vi "UpgradeFirmware_Main.vi"(8 "error in (no error)":errorcluster, 11 "DevInfo":T1={"Hostname"="", "IPAddress"="", "MAC"="", "SerialNum"="", "Model"="", "Status"="", "FW"="", "OSDesc"="", "ImgTitle"="", "ImgDesc"="", "ImgVer"="", "ImgID"="", "IP Address Request Mode"=1, "SubnetMask"="", "Gateway"="", "DNSServer"=""} {"IP Address Request Mode" items=["Static"=1, "DHCP/Link-Local"=2, "Link-Local Only"=4, "DHCP Only"=8]}) -> (0 "error out":errorcluster)   [LabVIEW 2021]
uses:
  TypeDefs/DevInfo.ctl
  TypeDefs/DeployImageStates.ctl
  TypeDefs/AppImageProperties.ctl
  TypeDefs/FPGA_Properties_Element.ctl
  <vilib>/Utility/config.llb/Read Key (String).vi
  <vilib>/Utility/config.llb/NI_LVConfig.lvlib
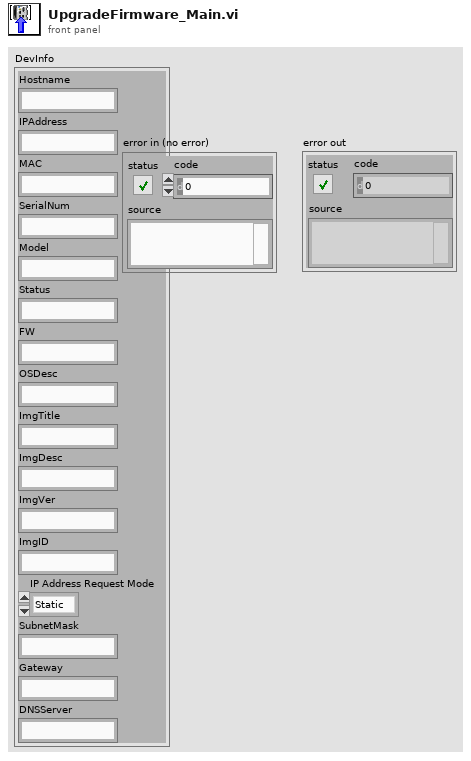
[diagram p1: front panel]
types:
  T1 = typedef "DevInfo.ctl" = cluster{"Hostname":string, "IPAddress":string, "MAC":string, "SerialNum":string, "Model":string, "Status":string, "FW":string, "OSDesc":string, "ImgTitle":string, "ImgDesc":string, "ImgVer":string, "ImgID":string, "IP Address Request Mode":i32, "SubnetMask":string, "Gateway":string, "DNSServer":string}
  T2 = typedef "AppImageProperties.ctl" = cluster{"Name":string, "Version":string, "Time":timestamp, "Description":string, "Key":string, "Chassis":string, "FPGA Properties":T3[], "Model":string, "Retrieve":string[], "Deploy":string[], "Installed Software":string[]}
  T3 = typedef "FPGA_Properties_Element.ctl" = cluster{"Resource Name":string, "Path":path}
  T4 = typedef "DeployImageStates.ctl" = enum16{"Select Image File", "Extract Image", "Display Image Info", "Deploy Image", "Clean Up", "Exit"}
  T5 = cluster{"Selected Image File":path, "AppImage Properties":T2}
  T6 = typedef "NI_LVConfig.lvlib/Config Data RefNum.ctl" = refnum<k1>
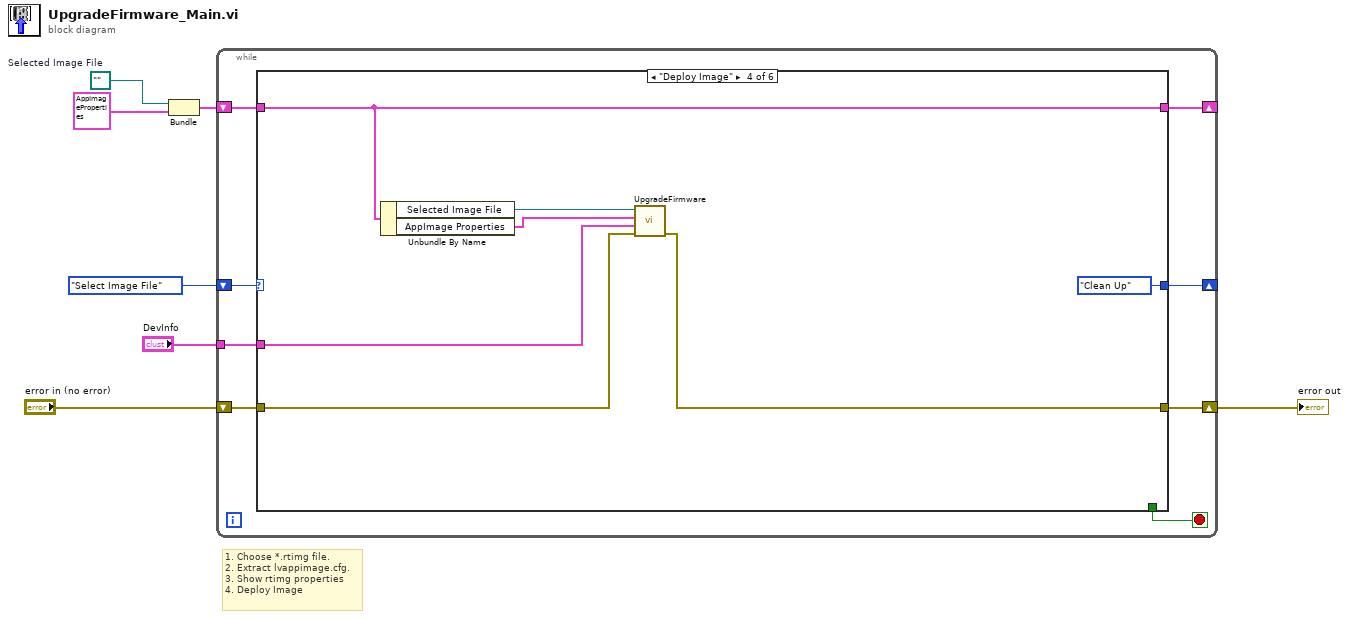
[diagram p0: block diagram]
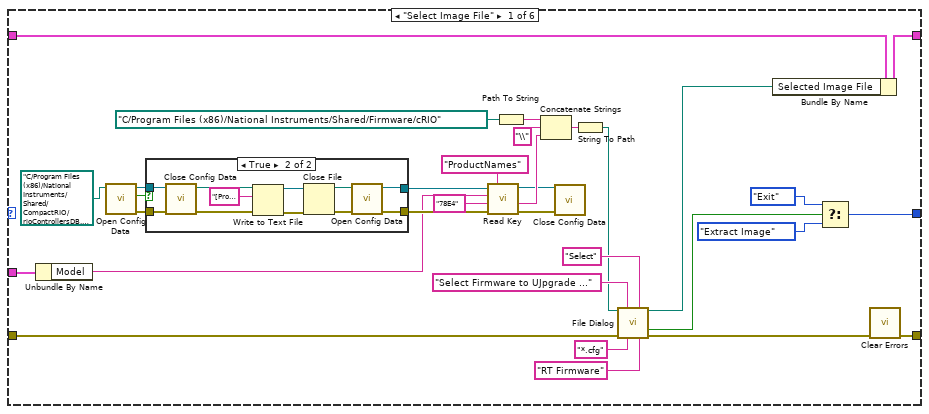
[diagram p2: hidden frame]
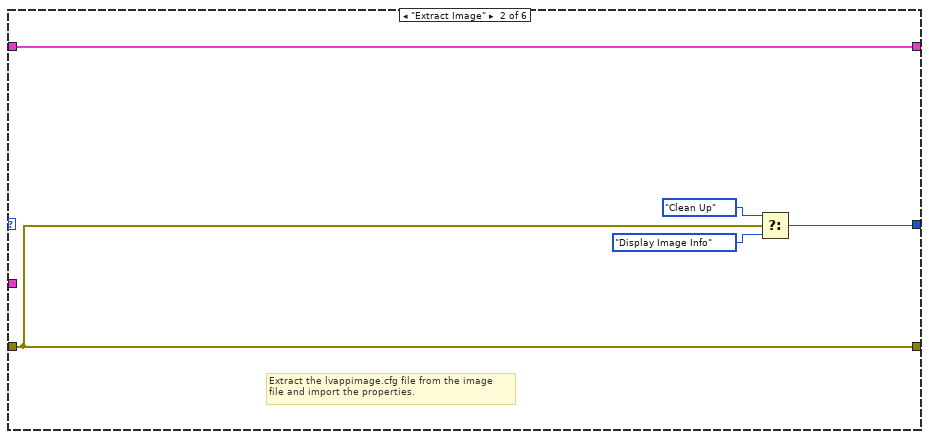
[diagram p4: hidden frame]
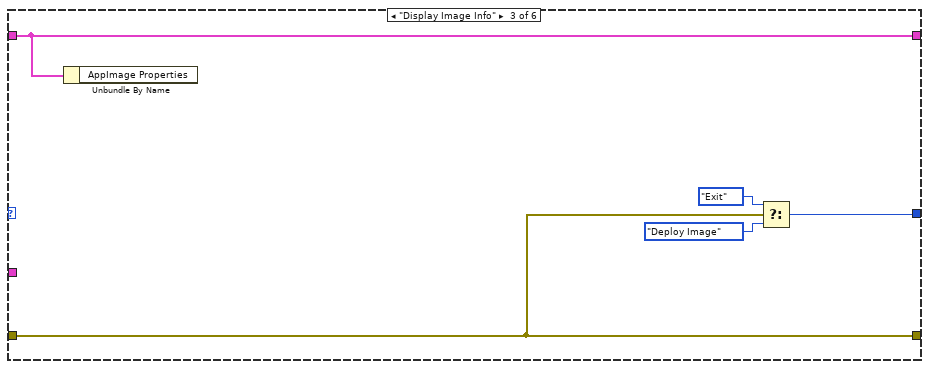
[diagram p5: hidden frame]
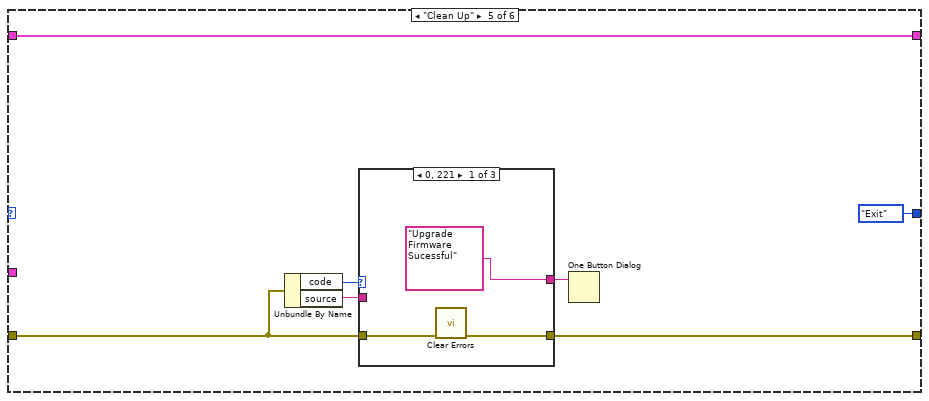
[diagram p6: hidden frame]
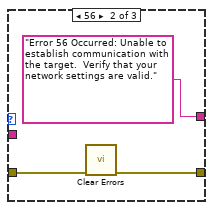
[diagram p7: hidden frame]
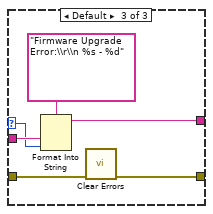
[diagram p8: hidden frame]
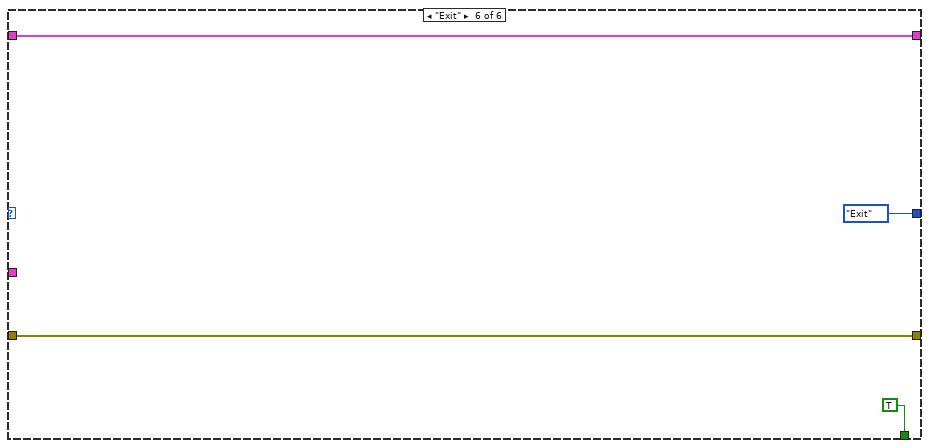
[diagram p9: hidden frame]
diagram:
  w4 = path ""  # Selected Image File
  # "1. Choose *.rtimg file.\n2. Extract lvappimage.cfg.\n3. Show rtimg properties\n4. Deploy Image"
  n1 = Bundle("Selected Image File"=w4, "AppImage Properties"=T2 {"Name"="", "Version"="", "Time"=timestamp(0 s since 1904-01-01), "Description"="", "Key"="", "Chassis"="", "FPGA Properties"=[], "Model"="", "Retrieve"=[], "Deploy"=[], "Installed Software"=[]}) -> (w3:T5)  [unwired: 1 in]
  n2 = while {
    shift-right: [w12] -> _
    shift-left: DeployImageStates."Select Image File" -> [w15]
    shift-right: [w13] -> w5
    shift-left: "error in (no error)" -> [w14]
    shift-right: [w10] -> _
    shift-left: w3 -> [w11]
    tunnel: "DevInfo" -> [w8]
    stop <- w9 stop-if-true
    n3 = case shown="\"Deploy Image\"" w15 {
      tunnel: w14 -> [w44 w65 w66 w72 w81 w98]
      tunnel: [w38 w65 w66 w71 w80 w98] -> w13
      tunnel: [w40 w61 w68 DeployImageStates."Clean Up" DeployImageStates."Exit" DeployImageStates."Exit"] -> w12
      tunnel: w11 -> [w34 w64 w67 w76 w79 w99]
      tunnel: [w37 w64 w67 w76 w79 w99] -> w10
      tunnel: [_ _ _ _ _ TRUE] -> w9
      tunnel: w8 -> [w17 _ _ w73 _ _]
      frame "Select Image File" {
        n4 = Unbundle By Name(w17) -> ("Model"=w16:string)
        n5 = call <vilib>:"Open Config Data.vi"("configuration file path"=path "C:/Program Files (x86)/National Instruments/Shared/CompactRIO/rioControllersDB.ini" ("start path")) -> ("error out"=w27:errorcluster, "file created?"=w25:bool, "refnum"=w26:T6)  [unwired: 8 in]
        n6 = case shown="True" w25 {
          tunnel: w26 -> [w49 w60]
          tunnel: w27 -> [w48 w59]
          tunnel: [w49 w54] -> w28
          tunnel: [w48 w50] -> w29
          frame False {
          }
          frame True {
            n7 = call <vilib>:"Close Config Data.vi"("error in (no error)"=w59, "refnum"=w60) -> ("error out"=w52:errorcluster, "file path"=w58:path)  [unwired: 8 in]
            n8 = Write to Text File(file (use dialog)=w58, text="[ProductNames]\nsbRIO-9601=7373\nsbRIO-9602=7373\nsbRIO-9611=7373\nsbRIO-9612=7373\nsbRIO-9631=7373\nsbRIO-9632=7373\nsbRIO-9641=7373\nsbRIO-9642=7373\nsbRIO-9605=758B\nsbRIO-9606=758B\nsbRIO-9623=758B\nsbRIO-9626=758B\nsbRIO-9633=758B\nsbRIO-9636=758B\nsbRIO-9651=775E\nsbRIO-9607=77D6\nsbRIO-9627=77D5\nsbRIO-9637=77D4\nsbRIO-9603=7A38\nsbRIO-9608=7A39\nsbRIO-9609=7A41\nsbRIO-9628=7A3A\nsbRIO-9629=7A43\nsbRIO-9638=7A3B\n\ncRIO-9002=705F\ncRIO-9004=705F\ncRIO-9012=718F\ncRIO-9014=7319\ncRIO-9022=73D2\ncRIO-9023=73D2\ncRIO-9024=7459\ncRIO-9025=7459\ncRIO-9030=7755\ncRIO-9031=774B\ncRIO-9032=7841\ncRIO-9033=7735\ncRIO-9034=774D\ncRIO-9035=77DB\ncRIO-9035 (Sync)=7875\ncRIO-9036=77DC\ncRIO-9037=7840\ncRIO-9038=77B9\ncRIO-9039=77DD\ncRIO-9039 (Sync)=7878\ncRIO-9040=78E3\ncRIO-9041=79D0\ncRIO-9042=78E8\ncRIO-9043=78E5\ncRIO-9045=78E4\ncRIO-9046=79CE\ncRIO-9047=78E9\ncRIO-9048=78B7\ncRIO-9048 (TPM)=78E7\ncRIO-9049=78EA\ncRIO-9053=79DD\ncRIO-9054=79DE\ncRIO-9055=7A2B\ncRIO-9056=79DF\ncRIO-9057=79E0\ncRIO-9058=7A2A\ncRIO-9072=71C7\ncRIO-9073=71C7\ncRIO-9074=729D\ncRIO-9075=7527\ncRIO-9076=7527\ncRIO-9081=753D\ncRIO-9082=753D\ncRIO-9081_$$=751A\ncRIO-9082_$$=751A\ncRIO-9063=7740\ncRIO-9064=7741\ncRIO-9065=7742\ncRIO-9066=7743\ncRIO-9067=7744\ncRIO-9068=76D6\n\nNI 9146=75C8\nNI 9147=774C\nNI 9148=74E8\nNI 9149=774E\n\nmyRIO-1900=762F\nmyRIO-1950=76D3\nroboRIO=76F2\nroboRIO 2.0=7AAE\nELVIS RIO CM=7885\nELVIS III=793C\n\ncRIO-9081_$$_$$=753D_2\ncRIO-9082_$$_$$=753D_2\n\n; lvRioProviderVersion is Major*1000000 + Minor*1000 + Update\n[LabVIEWSupportRemoved_lvRioProviderVersion]\ncRIO-9002=17000000\ncRIO-9004=17000000\ncRIO-9072=17000000\ncRIO-9012=19000000\ncRIO-9014=19000000\ncRIO-9022=20000000\ncRIO-9023=20000000\ncRIO-9024=20000000\ncRIO-9025=20000000\ncRIO-9072=20000000\ncRIO-9073=20000000\ncRIO-9074=20000000\ncRIO-9075=20000000\ncRIO-9076=20000000\ncRIO-9081=20000000\ncRIO-9082=20000000\ncRIO-9081_$$=20000000\ncRIO-9082_$$=20000000\ncRIO-9081_$$_$$=20000000\ncRIO-9082_$$_$$=20000000\nsbRIO-9601=20000000\nsbRIO-9602=20000000\nsbRIO-9611=20000000\nsbRIO-9612=20000000\nsbRIO-9631=20000000\nsbRIO-9632=20000000\nsbRIO-9641=20000000\nsbRIO-9642=20000000\nsbRIO-9605=20000000\nsbRIO-9606=20000000\nsbRIO-9623=20000000\nsbRIO-9626=20000000\nsbRIO-9633=20000000\nsbRIO-9636=20000000\nNI 9146=20000000\nNI 9148=20000000\n\n[7373]\nsupportChassisAddition_lvRioProviderVersion=14000000\nsupportedInLabVIEW_lvRioProviderVersion=13000000\nproductLine=sbRIO\npngIcon16=SingleBoardRIOController.png\npngWarningIcon16=SingleBoardRIOControllerWarning.png\noperatingSystem=vxworks\ncpuArchitecture=ppc\nmonolithic=true\nsupportsRsi_lvRioProviderVersion=13000000\n\n[758B]\nsupportChassisAddition_lvRioProviderVersion=14000000\nsupportedInLabVIEW_lvRioProviderVersion=13000000\nproductLine=sbRIO\npngIcon16=SingleBoardRIOController.png\npngWarningIcon16=SingleBoardRIOControllerWarning.png\noperatingSystem=vxworks\ncpuArchitecture=ppc\nmonolithic=true\nneedsDDPSwitches=true\nsupportsRsi_lvRioProviderVersion=13000000\n\n[705F]\nsupportChassisAddition_lvRioProviderVersion=14000000\nsupportedInLabVIEW_lvRioProviderVersion=13000000\nproductLine=cRIO\npngIcon16=CompactRIOController.png\npngWarningIcon16=CompactRIOControllerWarning.png\noperatingSystem=pharlap\ncpuArchitecture=x86\n\n[718F]\nsupportChassisAddition_lvRioProviderVersion=14000000\nsupportedInLabVIEW_lvRioProviderVersion=13000000\nproductLine=cRIO\npngIcon16=CompactRIOController.png\npngWarningIcon16=CompactRIOControllerWarning.png\noperatingSystem=vxworks\ncpuArchitecture=ppc\nsupportsRsi_lvRioProviderVersion=13000000\n\n[7319]\nsupportChassisAddition_lvRioProviderVersion=14000000\nsupportedInLabVIEW_lvRioProviderVersion=13000000\nproductLine=cRIO\npngIcon16=CompactRIOController.png\npngWarningIcon16=CompactRIOControllerWarning.png\noperatingSystem=vxworks\ncpuArchitecture=ppc\nsupportsRsi_lvRioProviderVersion=13000000\n\n[73D2]\nsupportChassisAddition_lvRioProviderVersion=14000000\nsupportedInLabVIEW_lvRioProviderVersion=13000000\nproductLine=cRIO\npngIcon16=CompactRIOController.png\npngWarningIcon16=CompactRIOControllerWarning.png\noperatingSystem=vxworks\ncpuArchitecture=ppc\nsupportsRsi_lvRioProviderVersion=13000000\n\n[7459]\nsupportChassisAddition_lvRioProviderVersion=14000000\nsupportedInLabVIEW_lvRioProviderVersion=13000000\nproductLine=cRIO\npngIcon16=CompactRIOController.png\npngWarningIcon16=CompactRIOControllerWarning.png\noperatingSystem=vxworks\ncpuArchitecture=ppc\nsupportsRsi_lvRioProviderVersion=13000000\n\n[7755]\nsupportChassisAddition_lvRioProviderVersion=14000000\nsupportedInLabVIEW_lvRioProviderVersion=14000000\nproductLine=cRIO\npngIcon16=CompactRIOController.png\npngWarningIcon16=CompactRIOControllerWarning.png\noperatingSystem=linux\ncpuArchitecture=x64\nmonolithic=true\nsupportsRsi_lvRioProviderVersion=14000000\n\n[774B]\nsupportChassisAddition_lvRioProviderVersion=14000000\nsupportedInLabVIEW_lvRioProviderVersion=14000000\nproductLine=cRIO\npngIcon16=CompactRIOController.png\npngWarningIcon16=CompactRIOControllerWarning.png\noperatingSystem=linux\ncpuArchitecture=x64\nmonolithic=true\nsupportsRsi_lvRioProviderVersion=14000000\n\n[7841]\nsupportChassisAddition_lvRioProviderVersion=15000000\nsupportedInLabVIEW_lvRioProviderVersion=15000000\nproductLine=cRIO\npngIcon16=CompactRIOController.png\npngWarningIcon16=CompactRIOControllerWarning.png\noperatingSystem=linux\ncpuArchitecture=x64\nmonolithic=true\nsupportsRsi_lvRioProviderVersion=15000000\n\n[7735]\nsupportChassisAddition_lvRioProviderVersion=14000000\nsupportedInLabVIEW_lvRioProviderVersion=14000000\nproductLine=cRIO\npngIcon16=CompactRIOController.png\npngWarningIcon16=CompactRIOControllerWarning.png\noperatingSystem=linux\ncpuArchitecture=x64\nmonolithic=true\nsupportsRsi_lvRioProviderVersion=14000000\n\n[774D]\nsupportChassisAddition_lvRioProviderVersion=14000000\nsupportedInLabVIEW_lvRioProviderVersion=14000000\nproductLine=cRIO\npngIcon16=CompactRIOController.png\npngWarningIcon16=CompactRIOControllerWarning.png\noperatingSystem=linux\ncpuArchitecture=x64\nmonolithic=true\nsupportsRsi_lvRioProviderVersion=14000000\n\n[77DB]\nsupportChassisAddition_lvRioProviderVersion=14005000\nsupportedInLabVIEW_lvRioProviderVersion=14005000\nproductLine=cRIO\npngIcon16=CompactRIOController.png\npngWarningIcon16=CompactRIOControllerWarning.png\noperatingSystem=linux\ncpuArchitecture=x64\nmonolithic=true\nsupportsRsi_lvRioProviderVersion=14005000\n\n[77DC]\nsupportChassisAddition_lvRioProviderVersion=14005000\nsupportedInLabVIEW_lvRioProviderVersion=14005000\nproductLine=cRIO\npngIcon16=CompactRIOController.png\npngWarningIcon16=CompactRIOControllerWarning.png\noperatingSystem=linux\ncpuArchitecture=x64\nmonolithic=true\nsupportsRsi_lvRioProviderVersion=14005000\n\n[7840]\nsupportChassisAddition_lvRioProviderVersion=15000000\nsupportedInLabVIEW_lvRioProviderVersion=15000000\nproductLine=cRIO\npngIcon16=CompactRIOController.png\npngWarningIcon16=CompactRIOControllerWarning.png\noperatingSystem=linux\ncpuArchitecture=x64\nmonolithic=true\nsupportsRsi_lvRioProviderVersion=15000000\n\n[77B9]\nsupportChassisAddition_lvRioProviderVersion=14000000\nsupportedInLabVIEW_lvRioProviderVersion=14000000\nproductLine=cRIO\npngIcon16=CompactRIOController.png\npngWarningIcon16=CompactRIOControllerWarning.png\noperatingSystem=linux\ncpuArchitecture=x64\nmonolithic=true\nsupportsRsi_lvRioProviderVersion=14000000\n\n[77DD]\nsupportChassisAddition_lvRioProviderVersion=14005000\nsupportedInLabVIEW_lvRioProviderVersion=14005000\nproductLine=cRIO\npngIcon16=CompactRIOController.png\npngWarningIcon16=CompactRIOControllerWarning.png\noperatingSystem=linux\ncpuArchitecture=x64\nmonolithic=true\nsupportsRsi_lvRioProviderVersion=14005000\n\n[78E3]\nsupportsTimeSync=true\nsupportChassisAddition_lvRioProviderVersion=17006000\nsupportedInLabVIEW_lvRioProviderVersion=17006000\nproductLine=cRIO\npngIcon16=CompactRIOController.png\npngWarningIcon16=CompactRIOControllerWarning.png\noperatingSystem=linux\ncpuArchitecture=x64\nmonolithic=true\nsupportsRsi_lvRioProviderVersion=17006000\nsupportsDaqMode_lvRioProviderVersion=17006000\n\n[79D0]\nsupportsTimeSync=true\nsupportChassisAddition_lvRioProviderVersion=17006000\nsupportedInLabVIEW_lvRioProviderVersion=17006000\nproductLine=cRIO\npngIcon16=CompactRIOController.png\npngWarningIcon16=CompactRIOControllerWarning.png\noperatingSystem=linux\ncpuArchitecture=x64\nmonolithic=true\nsupportsRsi_lvRioProviderVersion=17006000\nsupportsDaqMode_lvRioProviderVersion=17006000\n\n[79CE]\nsupportsTimeSync=true\nsupportChassisAddition_lvRioProviderVersion=17006000\nsupportedInLabVIEW_lvRioProviderVersion=17006000\nproductLine=cRIO\npngIcon16=CompactRIOController.png\npngWarningIcon16=CompactRIOControllerWarning.png\noperatingSystem=linux\ncpuArchitecture=x64\nmonolithic=true\nsupportsRsi_lvRioProviderVersion=17006000\nsupportsDaqMode_lvRioProviderVersion=17006000\n\n[78E8]\nsupportsTimeSync=true\nsupportChassisAddition_lvRioProviderVersion=17006000\nsupportedInLabVIEW_lvRioProviderVersion=17006000\nproductLine=cRIO\npngIcon16=CompactRIOController.png\npngWarningIcon16=CompactRIOControllerWarning.png\noperatingSystem=linux\ncpuArchitecture=x64\nmonolithic=true\nsupportsRsi_lvRioProviderVersion=17006000\nsupportsDaqMode_lvRioProviderVersion=17006000\n\n[78E5]\nsupportsTimeSync=true\nsupportChassisAddition_lvRioProviderVersion=17006000\nsupportedInLabVIEW_lvRioProviderVersion=17006000\nproductLine=cRIO\npngIcon16=CompactRIOController.png\npngWarningIcon16=CompactRIOControllerWarning.png\noperatingSystem=linux\ncpuArchitecture=x64\nmonolithic=true\nsupportsRsi_lvRioProviderVersion=17006000\nsupportsDaqMode_lvRioProviderVersion=17006000\n\n[78E4]\nsupportsTimeSync=true\nsupportChassisAddition_lvRioProviderVersion=17006000\nsupportedInLabVIEW_lvRioProviderVersion=17006000\nproductLine=cRIO\npngIcon16=CompactRIOController.png\npngWarningIcon16=CompactRIOControllerWarning.png\noperatingSystem=linux\ncpuArchitecture=x64\nmonolithic=true\nsupportsRsi_lvRioProviderVersion=17006000\nsupportsDaqMode_lvRioProviderVersion=17006000\n\n[78E9]\nsupportsTimeSync=true\nsupportChassisAddition_lvRioProviderVersion=17006000\nsupportedInLabVIEW_lvRioProviderVersion=17006000\nproductLine=cRIO\npngIcon16=CompactRIOController.png\npngWarningIcon16=CompactRIOControllerWarning.png\noperatingSystem=linux\ncpuArchitecture=x64\nmonolithic=true\nsupportsRsi_lvRioProviderVersion=17006000\nsupportsDaqMode_lvRioProviderVersion=17006000\n\n[78B7]\nsupportsTimeSync=true\nsupportChassisAddition_lvRioProviderVersion=17006000\nsupportedInLabVIEW_lvRioProviderVersion=17006000\nproductLine=cRIO\npngIcon16=CompactRIOController.png\npngWarningIcon16=CompactRIOControllerWarning.png\noperatingSystem=linux\ncpuArchitecture=x64\nmonolithic=true\nsupportsRsi_lvRioProviderVersion=17006000\nsupportsDaqMode_lvRioProviderVersion=17006000\n\n[78E7]\nsupportsTimeSync=true\nsupportChassisAddition_lvRioProviderVersion=18001000\nsupportedInLabVIEW_lvRioProviderVersion=18001000\nproductLine=cRIO\npngIcon16=CompactRIOController.png\npngWarningIcon16=CompactRIOControllerWarning.png\noperatingSystem=linux\ncpuArchitecture=x64\nmonolithic=true\ninvisibleToAddNewUnlessKeyEnabled=isTPMcRIOSupported\nsupportsRsi_lvRioProviderVersion=18001000\nsupportsDaqMode_lvRioProviderVersion=18001000\n\n[78EA]\nsupportsTimeSync=true\nsupportChassisAddition_lvRioProviderVersion=17006000\nsupportedInLabVIEW_lvRioProviderVersion=17006000\nproductLine=cRIO\npngIcon16=CompactRIOController.png\npngWarningIcon16=CompactRIOControllerWarning.png\noperatingSystem=linux\ncpuArchitecture=x64\nmonolithic=true\nsupportsRsi_lvRioProviderVersion=17006000\nsupportsDaqMode_lvRioProviderVersion=17006000\n\n[79DD]\nsupportsTimeSync=true\nsupportChassisAddition_lvRioProviderVersion=18000000\nsupportedInLabVIEW_lvRioProviderVersion=18000000\nproductLine=cRIO\npngIcon16=CompactRIOController.png\npngWarningIcon16=CompactRIOControllerWarning.png\noperatingSystem=linux\ncpuArchitecture=x64\nmonolithic=true\nsupportsRsi_lvRioProviderVersion=18000000\nsupportsDaqMode_lvRioProviderVersion=18000000\n\n[79DE]\nsupportsTimeSync=true\nsupportChassisAddition_lvRioProviderVersion=18000000\nsupportedInLabVIEW_lvRioProviderVersion=18000000\nproductLine=cRIO\npngIcon16=CompactRIOController.png\npngWarningIcon16=CompactRIOControllerWarning.png\noperatingSystem=linux\ncpuArchitecture=x64\nmonolithic=true\nsupportsRsi_lvRioProviderVersion=18000000\nsupportsDaqMode_lvRioProviderVersion=18000000\n\n[7A2B]\nsupportsTimeSync=true\nsupportChassisAddition_lvRioProviderVersion=19000000\nsupportedInLabVIEW_lvRioProviderVersion=19000000\nproductLine=cRIO\npngIcon16=CompactRIOController.png\npngWarningIcon16=CompactRIOControllerWarning.png\noperatingSystem=linux\ncpuArchitecture=x64\nmonolithic=true\nsupportsRsi_lvRioProviderVersion=19000000\nsupportsDaqMode_lvRioProviderVersion=19000000\n\n[79DF]\nsupportsTimeSync=true\nsupportChassisAddition_lvRioProviderVersion=18000000\nsupportedInLabVIEW_lvRioProviderVersion=18000000\nproductLine=cRIO\npngIcon16=CompactRIOController.png\npngWarningIcon16=CompactRIOControllerWarning.png\noperatingSystem=linux\ncpuArchitecture=x64\nmonolithic=true\nsupportsRsi_lvRioProviderVersion=18000000\nsupportsDaqMode_lvRioProviderVersion=18000000\n\n[79E0]\nsupportsTimeSync=true\nsupportChassisAddition_lvRioProviderVersion=18000000\nsupportedInLabVIEW_lvRioProviderVersion=18000000\nproductLine=cRIO\npngIcon16=CompactRIOController.png\npngWarningIcon16=CompactRIOControllerWarning.png\noperatingSystem=linux\ncpuArchitecture=x64\nmonolithic=true\nsupportsRsi_lvRioProviderVersion=18000000\nsupportsDaqMode_lvRioProviderVersion=18000000\n\n[7A2A]\nsupportsTimeSync=true\nsupportChassisAddition_lvRioProviderVersion=19000000\nsupportedInLabVIEW_lvRioProviderVersion=19000000\nproductLine=cRIO\npngIcon16=CompactRIOController.png\npngWarningIcon16=CompactRIOControllerWarning.png\noperatingSystem=linux\ncpuArchitecture=x64\nmonolithic=true\nsupportsRsi_lvRioProviderVersion=19000000\nsupportsDaqMode_lvRioProviderVersion=19000000\n\n[71C7]\nsupportChassisAddition_lvRioProviderVersion=14000000\nsupportedInLabVIEW_lvRioProviderVersion=13000000\nproductLine=cRIO\npngIcon16=CompactRIOController.png\npngWarningIcon16=CompactRIOControllerWarning.png\noperatingSystem=vxworks\ncpuArchitecture=ppc\nmonolithic=true\nsupportsRsi_lvRioProviderVersion=13000000\n\n[729D]\nsupportChassisAddition_lvRioProviderVersion=14000000\nsupportedInLabVIEW_lvRioProviderVersion=13000000\nproductLine=cRIO\npngIcon16=CompactRIOController.png\npngWarningIcon16=CompactRIOControllerWarning.png\noperatingSystem=vxworks\ncpuArchitecture=ppc\nmonolithic=true\nsupportsRsi_lvRioProviderVersion=13000000\n\n[7527]\nsupportChassisAddition_lvRioProviderVersion=14000000\nsupportedInLabVIEW_lvRioProviderVersion=13000000\nproductLine=cRIO\npngIcon16=CompactRIOController.png\npngWarningIcon16=CompactRIOControllerWarning.png\noperatingSystem=vxworks\ncpuArchitecture=ppc\nmonolithic=true\nsupportsRsi_lvRioProviderVersion=13000000\nneedsDDPSwitches=true\n\n[753D]\nsupportChassisAddition_lvRioProviderVersion=14000000\nsupportedInLabVIEW_lvRioProviderVersion=13000000\nproductLine=cRIO\npngIcon16=CompactRIOController.png\npngWarningIcon16=CompactRIOControllerWarning.png\noperatingSystem=pharlap\ncpuArchitecture=x86\nmonolithic=true\nsupportsMxiE=true\ninvisibleToAddNew=false\nsupportsRtSmpPalette=true\nsupportsRsi_lvRioProviderVersion=13000000\n\n[751A]\nsupportChassisAddition_lvRioProviderVersion=14000000\nsupportedInLabVIEW_lvRioProviderVersion=13000000\nproductLine=cRIO\npngIcon16=CompactRIOController.png\npngWarningIcon16=CompactRIOControllerWarning.png\noperatingSystem=pharlap\ncpuArchitecture=x86\nmonolithic=true\nsupportsMxiE=true\ninvisibleToAddNew=true\nsupportsRtSmpPalette=true\nsupportsRsi_lvRioProviderVersion=13000000\n\n[7740]\nsupportChassisAddition_lvRioProviderVersion=14005000\nsupportedInLabVIEW_lvRioProviderVersion=14005000\nproductLine=cRIO\npngIcon16=CompactRIOController.png\npngWarningIcon16=CompactRIOControllerWarning.png\noperatingSystem=linux\ncpuArchitecture=arm\nmonolithic=true\nsupportsRsi_lvRioProviderVersion=14005000\n\n[7741]\nsupportChassisAddition_lvRioProviderVersion=14005000\nsupportedInLabVIEW_lvRioProviderVersion=14005000\nproductLine=cRIO\npngIcon16=CompactRIOController.png\npngWarningIcon16=CompactRIOControllerWarning.png\noperatingSystem=linux\ncpuArchitecture=arm\nmonolithic=true\nsupportsRsi_lvRioProviderVersion=14005000\n\n[7742]\nsupportChassisAddition_lvRioProviderVersion=14005000\nsupportedInLabVIEW_lvRioProviderVersion=14005000\nproductLine=cRIO\npngIcon16=CompactRIOController.png\npngWarningIcon16=CompactRIOControllerWarning.png\noperatingSystem=linux\ncpuArchitecture=arm\nmonolithic=true\nsupportsRsi_lvRioProviderVersion=14005000\n\n[7743]\nsupportChassisAddition_lvRioProviderVersion=14000000\nsupportedInLabVIEW_lvRioProviderVersion=14000000\nproductLine=cRIO\npngIcon16=CompactRIOController.png\npngWarningIcon16=CompactRIOControllerWarning.png\noperatingSystem=linux\ncpuArchitecture=arm\nmonolithic=true\nsupportsRsi_lvRioProviderVersion=14000000\n\n[7744]\nsupportChassisAddition_lvRioProviderVersion=14000000\nsupportedInLabVIEW_lvRioProviderVersion=14000000\nproductLine=cRIO\npngIcon16=CompactRIOController.png\npngWarningIcon16=CompactRIOControllerWarning.png\noperatingSystem=linux\ncpuArchitecture=arm\nmonolithic=true\nsupportsRsi_lvRioProviderVersion=14000000\n\n[76D6]\nsupportChassisAddition_lvRioProviderVersion=14000000\nsupportedInLabVIEW_lvRioProviderVersion=13000000\nproductLine=cRIO\npngIcon16=CompactRIOController.png\npngWarningIcon16=CompactRIOControllerWarning.png\noperatingSystem=linux\ncpuArchitecture=arm\nmonolithic=true\nsupportsRsi_lvRioProviderVersion=13000000\n\n[74E8]\nsupportChassisAddition_lvRioProviderVersion=14000000\nsupportedInLabVIEW_lvRioProviderVersion=13000000\nproductLine=enetRIO\npngIcon16=cRIONonRTController.png\npngWarningIcon16=cRIONonRTControllerWarning.png\noperatingSystem=vxworks\ncpuArchitecture=ppc\nmonolithic=true\nsupportsRsi_lvRioProviderVersion=13000000\n\n[75C8]\nsupportChassisAddition_lvRioProviderVersion=14000000\nsupportedInLabVIEW_lvRioProviderVersion=13000000\nproductLine=enetRIO\npngIcon16=cRIONonRTController.png\npngWarningIcon16=cRIONonRTControllerWarning.png\noperatingSystem=vxworks\ncpuArchitecture=ppc\nmonolithic=true\nsupportsRsi_lvRioProviderVersion=13000000\nneedsDDPSwitches=true\ndialogModeForDDPSwitchesInt=1\n\n[762F]\nsupportChassisAddition_lvRioProviderVersion=14000000\nsupportedInLabVIEW_lvRioProviderVersion=13000000\nproductLine=myRIO\npngIcon16=EnclosedMyRIOController.png\npngWarningIcon16=EnclosedMyRIOControllerWarning.png\noperatingSystem=linux\ncpuArchitecture=arm\nmonolithic=true\nsupportsRsi_lvRioProviderVersion=13000000\n\n[76F2]\nsupportChassisAddition_lvRioProviderVersion=15000000\nsupportedInLabVIEW_lvRioProviderVersion=14000000\nproductLine=roboRIO\npngIcon16=RoboRIOController.png\npngWarningIcon16=RoboRIOControllerWarning.png\noperatingSystem=linux\ncpuArchitecture=arm\nmonolithic=true\nsupportsRsi_lvRioProviderVersion=14000000\n\n[7AAE]\nsupportChassisAddition_lvRioProviderVersion=20060000\nsupportedInLabVIEW_lvRioProviderVersion=20060000\nproductLine=roboRIO\npngIcon16=RoboRIOController.png\npngWarningIcon16=RoboRIOControllerWarning.png\noperatingSystem=linux\ncpuArchitecture=arm\nmonolithic=true\nsupportsRsi_lvRioProviderVersion=20060000\n\n[76D3]\nsupportChassisAddition_lvRioProviderVersion=14000000\nsupportedInLabVIEW_lvRioProviderVersion=13000000\nproductLine=myRIO\npngIcon16=SingleBoardMyRIOController.png\npngWarningIcon16=SingleBoardMyRIOControllerWarning.png\noperatingSystem=linux\ncpuArchitecture=arm\nmonolithic=true\nMAXIconInt=105\nsupportsRsi_lvRioProviderVersion=13000000\n\n[753D_2]\nsupportChassisAddition_lvRioProviderVersion=14000000\nsupportedInLabVIEW_lvRioProviderVersion=13000000\nproductLine=cRIOwindows\npngIcon16=CompactRIOController.png\npngWarningIcon16=CompactRIOControllerWarning.png\noperatingSystem=windows\ncpuArchitecture=x86\nmonolithic=true\nsupportsMxiE=true\n\n[774C]\nsupportChassisAddition_lvRioProviderVersion=14005000\nsupportedInLabVIEW_lvRioProviderVersion=14005000\nproductLine=enetRIO\npngIcon16=cRIONonRTController.png\npngWarningIcon16=cRIONonRTControllerWarning.png\noperatingSystem=linux\ncpuArchitecture=arm\nmonolithic=true\nsupportsRsi_lvRioProviderVersion=14005000\n\n[775E]\nsupportChassisAddition_lvRioProviderVersion=14000000\nsupportedInLabVIEW_lvRioProviderVersion=14000000\nproductLine=sbRIO\npngIcon16=SingleBoardRIOController.png\npngWarningIcon16=SingleBoardRIOControllerWarning.png\noperatingSystem=linux\ncpuArchitecture=arm\nmonolithic=true\nsupportsRsi_lvRioProviderVersion=14000000\n\n[774E]\nsupportChassisAddition_lvRioProviderVersion=14000000\nsupportedInLabVIEW_lvRioProviderVersion=14000000\nproductLine=enetRIO\npngIcon16=cRIONonRTController.png\npngWarningIcon16=cRIONonRTControllerWarning.png\noperatingSystem=linux\ncpuArchitecture=arm\nmonolithic=true\nsupportsRsi_lvRioProviderVersion=14000000\n\n[77D6]\nsupportChassisAddition_lvRioProviderVersion=15000000\nsupportedInLabVIEW_lvRioProviderVersion=15000000\nproductLine=sbRIO\npngIcon16=SingleBoardRIOController.png\npngWarningIcon16=SingleBoardRIOControllerWarning.png\noperatingSystem=linux\ncpuArchitecture=arm\nmonolithic=true\nsupportsRsi_lvRioProviderVersion=15000000\n\n[77D5]\nsupportChassisAddition_lvRioProviderVersion=15000000\nsupportedInLabVIEW_lvRioProviderVersion=15000000\nproductLine=sbRIO\npngIcon16=SingleBoardRIOController.png\npngWarningIcon16=SingleBoardRIOControllerWarning.png\noperatingSystem=linux\ncpuArchitecture=arm\nmonolithic=true\nsupportsRsi_lvRioProviderVersion=15000000\n\n[77D4]\nsupportChassisAddition_lvRioProviderVersion=15000000\nsupportedInLabVIEW_lvRioProviderVersion=15000000\nproductLine=sbRIO\npngIcon16=SingleBoardRIOController.png\npngWarningIcon16=SingleBoardRIOControllerWarning.png\noperatingSystem=linux\ncpuArchitecture=arm\nmonolithic=true\nsupportsRsi_lvRioProviderVersion=15000000\n\n[7875]\nsupportsTimeSync=true\nsupportChassisAddition_lvRioProviderVersion=15005000\nsupportedInLabVIEW_lvRioProviderVersion=15005000\nproductLine=cRIO\npngIcon16=CompactRIOController.png\npngWarningIcon16=CompactRIOControllerWarning.png\noperatingSystem=linux\ncpuArchitecture=x64\nmonolithic=true\nsupportsRsi_lvRioProviderVersion=15005000\n\n[7878]\nsupportsTimeSync=true\nsupportChassisAddition_lvRioProviderVersion=15005000\nsupportedInLabVIEW_lvRioProviderVersion=15005000\nproductLine=cRIO\npngIcon16=CompactRIOController.png\npngWarningIcon16=CompactRIOControllerWarning.png\noperatingSystem=linux\ncpuArchitecture=x64\nmonolithic=true\nsupportsRsi_lvRioProviderVersion=15005000\n\n[7885]\nsupportChassisAddition_lvRioProviderVersion=16000000\nsupportedInLabVIEW_lvRioProviderVersion=16000000\nproductLine=elvisRIOcm\npngIcon16=ElvisRIOController.png\npngWarningIcon16=ElvisRIOControllerWarning.png\noperatingSystem=linux\ncpuArchitecture=arm\nmonolithic=true\nsupportsRsi_lvRioProviderVersion=16000000\n\n[793C]\nsupportChassisAddition_lvRioProviderVersion=18000000\nsupportedInLabVIEW_lvRioProviderVersion=18000000\nproductLine=elvisRIOcm\npngIcon16=ElvisRIOController.png\npngWarningIcon16=ElvisRIOControllerWarning.png\noperatingSystem=linux\ncpuArchitecture=arm\nmonolithic=true\nsupportsElvisIIIPalette=true\nsupportsRsi_lvRioProviderVersion=18000000\n\n[7A38]\nsupportsTimeSync=true\nsupportChassisAddition_lvRioProviderVersion=19001000\nsupportedInLabVIEW_lvRioProviderVersion=19001000\nproductLine=sbRIO\npngIcon16=SingleBoardRIOController.png\npngWarningIcon16=SingleBoardRIOControllerWarning.png\noperatingSystem=linux\ncpuArchitecture=x64\nmonolithic=true\nsupportsRsi_lvRioProviderVersion=19001000\nsupportsDaqMode_lvRioProviderVersion=19001000\n\n[7A39]\nsupportsTimeSync=true\nsupportChassisAddition_lvRioProviderVersion=19001000\nsupportedInLabVIEW_lvRioProviderVersion=19001000\nproductLine=sbRIO\npngIcon16=SingleBoardRIOController.png\npngWarningIcon16=SingleBoardRIOControllerWarning.png\noperatingSystem=linux\ncpuArchitecture=x64\nmonolithic=true\nsupportsRsi_lvRioProviderVersion=19001000\nsupportsDaqMode_lvRioProviderVersion=19001000\n\n[7A41]\nsupportsTimeSync=true\nsupportChassisAddition_lvRioProviderVersion=19001000\nsupportedInLabVIEW_lvRioProviderVersion=19001000\nproductLine=sbRIO\npngIcon16=SingleBoardRIOController.png\npngWarningIcon16=SingleBoardRIOControllerWarning.png\noperatingSystem=linux\ncpuArchitecture=x64\nmonolithic=true\nsupportsRsi_lvRioProviderVersion=19001000\nsupportsDaqMode_lvRioProviderVersion=19001000\n\n[7A3A]\nsupportsTimeSync=true\nsupportChassisAddition_lvRioProviderVersion=19001000\nsupportedInLabVIEW_lvRioProviderVersion=19001000\nproductLine=sbRIO\npngIcon16=SingleBoardRIOController.png\npngWarningIcon16=SingleBoardRIOControllerWarning.png\noperatingSystem=linux\ncpuArchitecture=x64\nmonolithic=true\nsupportsRsi_lvRioProviderVersion=19001000\nsupportsDaqMode_lvRioProviderVersion=19001000\n\n[7A43]\nsupportsTimeSync=true\nsupportChassisAddition_lvRioProviderVersion=19001000\nsupportedInLabVIEW_lvRioProviderVersion=19001000\nproductLine=sbRIO\npngIcon16=SingleBoardRIOController.png\npngWarningIcon16=SingleBoardRIOControllerWarning.png\noperatingSystem=linux\ncpuArchitecture=x64\nmonolithic=true\nsupportsRsi_lvRioProviderVersion=19001000\nsupportsDaqMode_lvRioProviderVersion=19001000\n\n[7A3B]\nsupportsTimeSync=true\nsupportChassisAddition_lvRioProviderVersion=19001000\nsupportedInLabVIEW_lvRioProviderVersion=19001000\nproductLine=sbRIO\npngIcon16=SingleBoardRIOController.png\npngWarningIcon16=SingleBoardRIOControllerWarning.png\noperatingSystem=linux\ncpuArchitecture=x64\nmonolithic=true\nsupportsRsi_lvRioProviderVersion=19001000\nsupportsDaqMode_lvRioProviderVersion=19001000\n", error in=w52) -> (refnum out=w56:refnum<file>, error out=w53:errorcluster)  [unwired: 1 in, 1 out]
            n9 = Close File(refnum=w56, error in=w53) -> (path=w55:path, error out=w51:errorcluster)
            n10 = call <vilib>:"Open Config Data.vi"("error in (no error)"=w51, "configuration file path"=w55) -> ("error out"=w50:errorcluster, "refnum"=w54:T6)  [unwired: 7 in, 1 out]
          }
        }
        n11 = call-poly <vilib>:"Read Key.vi"("section"="ProductNames", "error in (no error)"=w29, "default value"="78E4", "key"=w16, "refnum"=w28) -> ("error out"=w31:errorcluster, "value"=w33:string, "refnum out"=w30:T6)  [unwired: 3 in, 1 out]
        n12 = Path To String(path=path "C:/Program Files (x86)/National Instruments/Shared/Firmware/cRIO" ("start path")) -> (string=w32:string)
        n13 = Concatenate Strings(w32, "\\" ("string"), w33) -> (w18:string)
        n14 = call <vilib>:"Close Config Data.vi"("error in (no error)"=w31, "refnum"=w30) -> ()  [unwired: 8 in, 2 out]
        n15 = String To Path(string=w18) -> (path=w20:path)
        n16 = call "File Dialog"("start path"=w20, "prompt"="Select Firmware to UJpgrade ...", "button label"="Select" ("prompt"), "error in"=w44, "pattern (all files)"="*.cfg", "pattern label"="RT Firmware") -> ("selected path"=w36:path, "cancelled"=w41:bool, "error out"=w39:errorcluster)  [unwired: 6 in, 1 out]
        n17 = Bundle By Name(cluster=w34, "Selected Image File"=w36) -> (w37:T5)
        n18 = Select(t=DeployImageStates."Exit", s=w41, f=DeployImageStates."Extract Image") -> (s? t:f=w40:T4)
        n19 = call <vilib>:"Clear Errors.vi"("error in (no error)"=w39) -> ("error out"=w38:errorcluster)  [unwired: 5 in, 1 out]
      }
      frame "Extract Image" {
        # "Extract the lvappimage.cfg file from the image\nfile and import the properties."
        n20 = Select(t=DeployImageStates."Clean Up", s=w65, f=DeployImageStates."Display Image Info") -> (s? t:f=w61:T4)
      }
      frame "Display Image Info" {
        n21 = Unbundle By Name(w67) -> ()  [unwired: 1 out]
        n22 = Select(t=DeployImageStates."Exit", s=w66, f=DeployImageStates."Deploy Image") -> (s? t:f=w68:T4)
      }
      frame "Deploy Image" {
        n23 = Unbundle By Name(w76) -> ("Selected Image File"=w75:path, "AppImage Properties"=w74:T2)
        n24 = call "UpgradeFirmware.vi"("error in (no error)"=w72, "DevInfo"=w73, "AppImage Properties"=w74, "Selected Image File"=w75) -> ("error out"=w71:errorcluster)  [unwired: 7 in]
      }
      frame "Clean Up" {
        n25 = Unbundle By Name(w81) -> ("code"=w83:i32, "source"=w84:string)
        n26 = case shown="0, 221" w83 {
          selector: w83 -> [_ _ w93]
          tunnel: w84 -> [_ _ w96]
          tunnel: ["Upgrade Firmware Sucessful" ("source") "Error 56 Occurred: Unable to establish communication with the target.  Verify that your network settings are valid." ("source") w95] -> w82
          tunnel: [w85 w88 w91] -> w80
          tunnel: w81 -> [w86 w89 w92]
          frame 0, 221 {
            n27 = call <vilib>:"Clear Errors.vi"("error in (no error)"=w86) -> ("error out"=w85:errorcluster)  [unwired: 5 in, 1 out]
          }
          frame 56 {
            n28 = call <vilib>:"Clear Errors.vi"("error in (no error)"=w89) -> ("error out"=w88:errorcluster)  [unwired: 5 in, 1 out]
          }
          frame Default {
            n29 = Format Into String(format string="Firmware Upgrade  Error:\\r\\n %s - %d", w96, w93) -> (resulting string=w95:string)  [unwired: 2 in, 1 out]
            n30 = call <vilib>:"Clear Errors.vi"("error in (no error)"=w92) -> ("error out"=w91:errorcluster)  [unwired: 5 in, 1 out]
          }
        }
        n31 = One Button Dialog(message=w82) -> ()  [unwired: 2 out]
      }
      frame "Exit" {
      }
    }
  }
  "error out" <- w5
